vi "Begin.vi"(8 "error in":errorcluster) -> (0 "error out":errorcluster)   [LabVIEW 2018]
doc: "Called before other user functions, this VI is expected to open initial I/O refnums, load in file data, and do all program initialization. Notice that the <B>error out</B> terminal is simply used for data flow. Wiring it to other structures or subVIs ensures that this VI runs first."
uses:
  <vilib>/Rock Robotics/WPI/DriverStation/WPI_DriverStationRobotMode2.ctl
  <vilib>/Rock Robotics/WPI/Joystick/WPI_JoystickDeviceEnum.ctl
  <vilib>/Rock Robotics/SystemInterfaces/DIO/FPGA_DIORelayChannel.ctl
  <vilib>/Rock Robotics/WPI/Relay/WPI_RelayDirection.ctl
  <vilib>/Rock Robotics/SystemInterfaces/AI/FPGA_AIChannel.ctl
  <vilib>/Rock Robotics/SystemInterfaces/DIO/FPGA_DIOChannel.ctl
  GP_states.ctl
  Robot Global Data.vi
  <vilib>/Rock Robotics/Network Tables/NT Write String Array.vi
  <vilib>/Rock Robotics/WPI/RobotDrive/WPI_RobotDriveOpen4MotorWithExistingMotors.vi
  drivers/ADIS16470 IMU/ADIS16470_IMU.lvlib
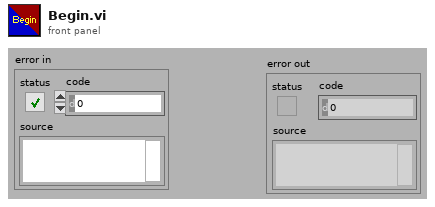
[diagram p1: front panel]
types:
  T1 = typedef "GP_states.ctl" = enum16{"Home", "AutoHome", "Hatch", "Ground"}
  T2 = enum16{"FollowerType_PercentOutput", "FollowerType_AuxOutput1"}
  T3 = typedef "FPGA_DIORelayChannel.ctl" = enum8{"Relay 0", "Relay 1", "Relay 2", "Relay 3", "Invalid"}
  T4 = typedef "WPI_RelayDirection.ctl" = enum16{"Both directions", "Forward only", "Reverse only"}
  T5 = typedef "FPGA_DIOChannel.ctl" = enum8{"DIO 0", "DIO 1", "DIO 2", "DIO 3", "DIO 4", "DIO 5", "DIO 6", "DIO 7", "DIO 8", "DIO 9", "DIO MXP 0", "DIO MXP 1", "DIO MXP 2", "DIO MXP 3", "DIO MXP 4", "DIO MXP 5", "DIO MXP 6", "DIO MXP 7", "DIO MXP 8", "DIO MXP 9", "DIO MXP 10", "DIO MXP 11", "DIO MXP 12", "DIO MXP 13", "DIO MXP 14", "DIO MXP 15", "SPI Port CS1", "SPI Port CS2", "SPI Port CS3", "SPI Port MISO", "SPI Port MOSI", "Invalid"}
  T6 = typedef "FPGA_AIChannel.ctl" = enum8{"AI 0", "AI 1", "AI 2", "AI 3", "AI MXP 0", "AI MXP 1", "AI MXP 2", "AI MXP 3", "Invalid"}
  T7 = typedef "WPI_JoystickDeviceEnum.ctl" = enum16{"USB 0", "USB 1", "USB 2", "USB 3", "USB 4", "USB 5"}
  T8 = typedef "WPI_DriverStationRobotMode2.ctl" = enum16{"Autonomous Disabled", "Autonomous Enabled", "Teleop Disabled", "Teleop Enabled", "Disconnected", "Finish", "Test Disabled", "Test Enabled", "Emergency Stopped"}
  T9 = typedef "WPI_MotorControlDeviceRef.ctl" = cluster{"DeviceStatus":errorcluster, "Type":T10, "PWM":cluster{"PWM Channel":T11, "DeadBand":T12}, "CAN":cluster{"Device Number":u8, "SetOutput VI Ref":variant, "GetOutput VI Ref":variant, "Enable VI Ref":variant, "Disable VI Ref":variant, "Data":variant}, "Invert":bool, "DIO PWM":cluster{"PWM \"Enable\" Channel":T11, "DIOChannel":T5, "PWM Rate":dbl}}
  T10 = typedef "WPI_MotorControlType.ctl" = enum16{"PWM", "CAN", "DIO PWM"}
  T11 = typedef "FPGA_DIOPWMChannel.ctl" = enum8{"PWM 0", "PWM 1", "PWM 2", "PWM 3", "PWM 4", "PWM 5", "PWM 6", "PWM 7", "PWM 8", "PWM 9", "PWM MXP 0", "PWM MXP 1", "PWM MXP 2", "PWM MXP 3", "PWM MXP 4", "PWM MXP 5", "PWM MXP 6", "PWM MXP 7", "PWM MXP 8", "PWM MXP 9", "Invalid"}
  T12 = typedef "WPI_PWMDeadband.ctl" = cluster{"Name":string, "maxPositivePwm":i32, "minPositivePwm":i32, "centerPwm":i32, "maxNegativePwm":i32, "minNegativePwm":i32, "angularRange":u16}
  T13 = typedef "WPI_JoystickDevRef.ctl" = cluster{"Device":T7}
  T14 = typedef "ADIS16470_IMU.lvlib/ADI_IMU_ADIS16470_IMUDevRef.ctl" = cluster{"DevStatus":errorcluster, "Handle":i32, "SPI Bus":T15, "Device Found":bool, "Device Ready":bool, "Serial":u16, "Bytes Per Sample":u16, "Calibrate On Open?":bool}
  T15 = typedef "spi_bus.ctl" = enum16{"SPI On-Board, CS0", "SPI On-Board, CS1", "SPI On-Board, CS2", "SPI On-Board, CS3", "SPI MXP", "Invalid"}
  T16 = typedef "WPI_RobotDriveDevRef.ctl" = cluster{"DevStatus":errorcluster, "Motors[]":T9[], "Square Inputs":bool, "Max Output":dbl}
  T17 = typedef "WPI_RelayDevRef.ctl" = cluster{"DevStatus":errorcluster, "Relay Channel":T3, "Relay Direction":T4}
  T18 = typedef "WPI_PotentiometerDevRef.ctl" = cluster{"DevStatus":errorcluster, "Analog Channel":T6, "Invert Output":bool}
  T19 = typedef "WPI_DigitalInputDevRef.ctl" = cluster{"DevStatus":errorcluster, "DIO Channel":T5}
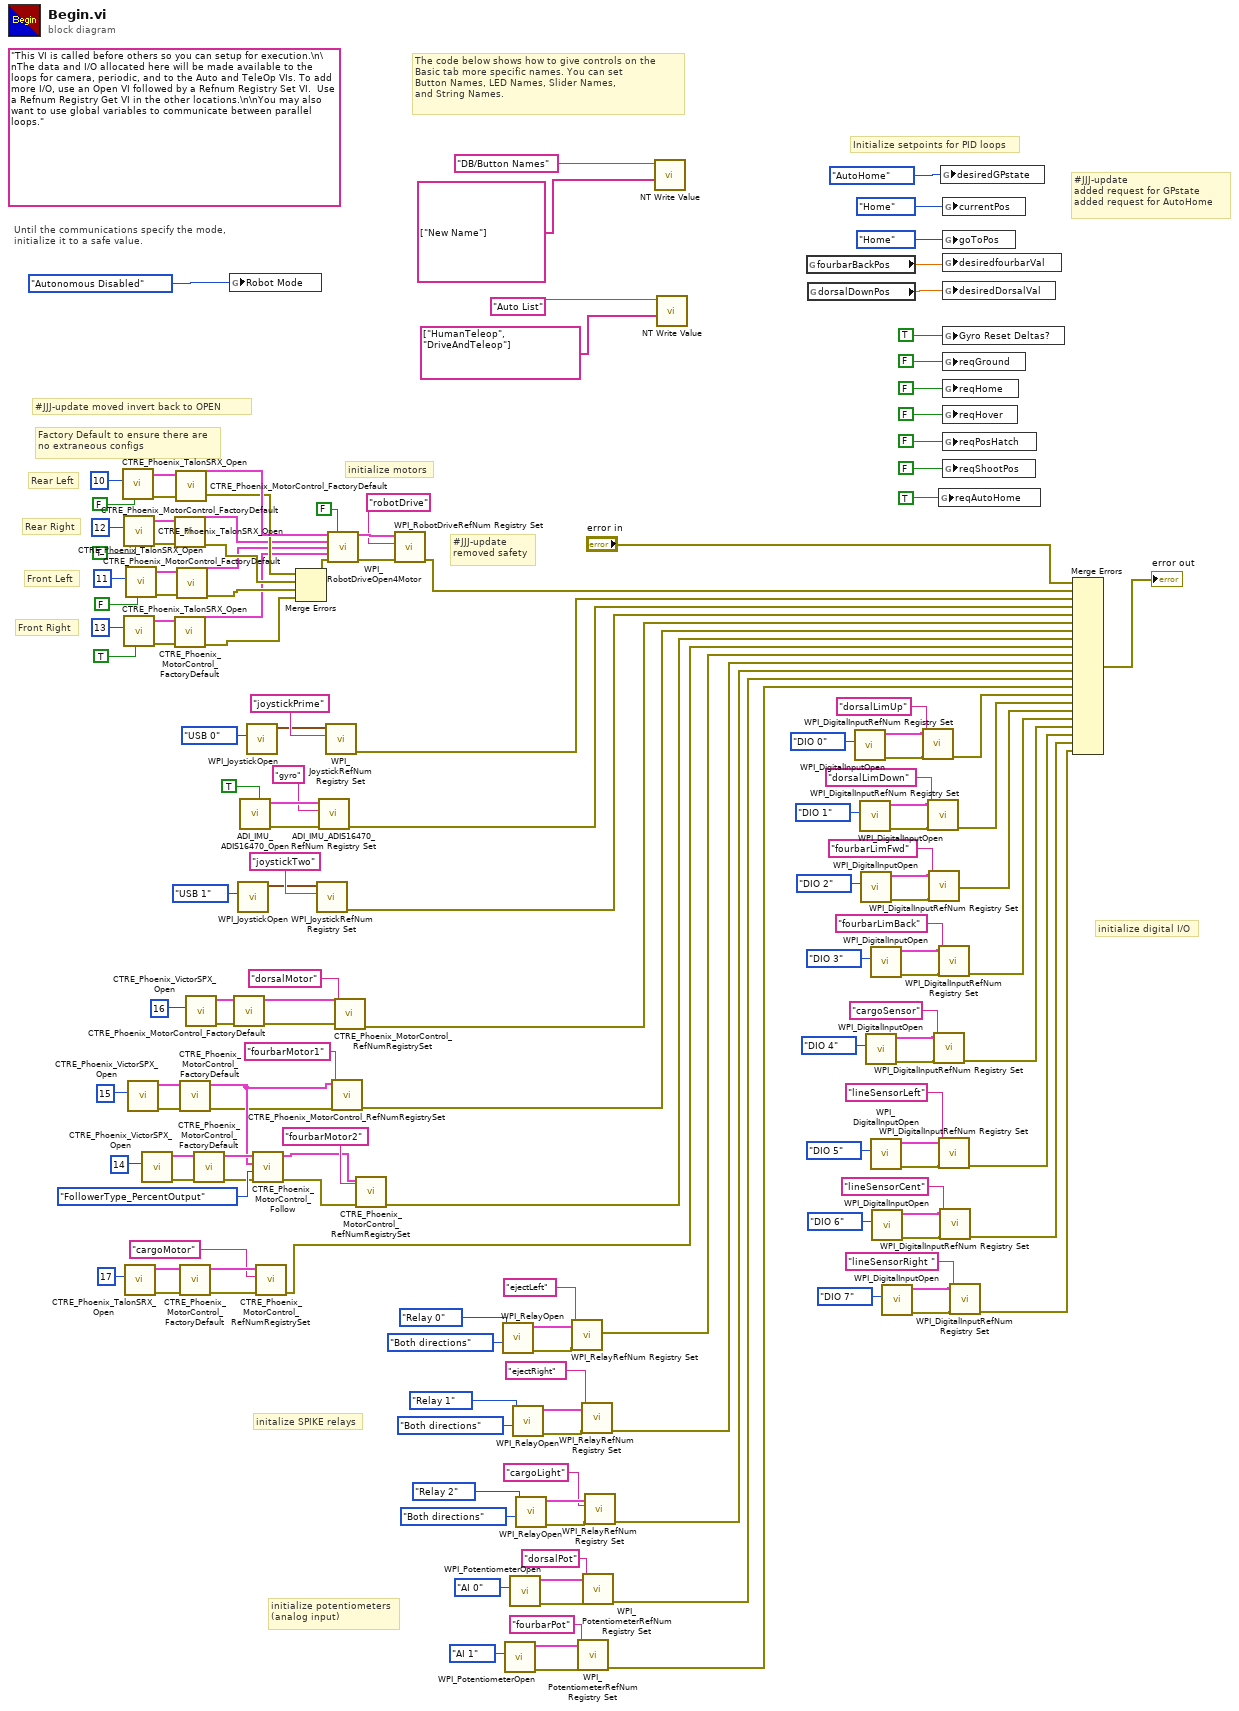
[diagram p0: block diagram]
diagram:
  (unwired) "This VI is called before others so you can setup for execution.\n\nThe data and I/O allocated here will be made available to the loops for camera, periodic, and to the Auto and TeleOp VIs. To add more I/O, use an Open VI followed by a Refnum Registry Set VI.  Use a Refnum Registry Get VI in the other locations.\n\nYou may also want to use global variables to communicate between parallel loops."
  # "#JJJ-update\nadded request for GPstate\nadded request for AutoHome"
  # "#JJJ-update\nremoved safety"
  # "#JJJ-update moved invert back to OPEN"
  # "Initialize setpoints for PID loops"
  # "initialize digital I/O"
  # "initialize potentiometers\n(analog input)"
  # "initalize SPIKE relays"
  # "Factory Default to ensure there are\nno extraneous configs"
  # "Front Right"
  # "Front Left"
  # "Rear Right"
  # "Rear Left"
  # "The code below shows how to give controls on the\nBasic tab more specific names. You can set\nButton Names, LED Names, Slider Names,\nand String Names."
  # "Until the communications specify the mode,\ninitialize it to a safe value."
  # "initialize motors"
  n1 = call <vilib>:"CTRE_Phoenix_TalonSRX_Open.vi"("Invert"=FALSE ("Invert?"), "Device Number"=u8 10) -> ("error out"=w144:errorcluster, "CAN Talon SRX Ref"=w145:T9)  [unwired: 8 in]
  n2 = call <vilib>:"CTRE_Phoenix_TalonSRX_Open.vi"("Invert"=TRUE ("Invert?"), "Device Number"=u8 12) -> ("error out"=w141:errorcluster, "CAN Talon SRX Ref"=w140:T9)  [unwired: 8 in]
  n3 = call <vilib>:"CTRE_Phoenix_TalonSRX_Open.vi"("Invert"=TRUE ("Invert?"), "Device Number"=u8 13) -> ("error out"=w135:errorcluster, "CAN Talon SRX Ref"=w134:T9)  [unwired: 8 in]
  n4 = call <vilib>:"CTRE_Phoenix_TalonSRX_Open.vi"("Device Number"=u8 17) -> ("error out"=w42:errorcluster, "CAN Talon SRX Ref"=w41:T9)  [unwired: 9 in]
  n5 = call <vilib>:"CTRE_Phoenix_TalonSRX_Open.vi"("Invert"=FALSE ("Invert?"), "Device Number"=u8 11) -> ("error out"=w136:errorcluster, "CAN Talon SRX Ref"=w137:T9)  [unwired: 8 in]
  n6 = call <vilib>:"CTRE_Phoenix_VictorSPX_Open.vi"("Device Number"=u8 15) -> ("error out"=w39:errorcluster, "CAN Talon SRX Ref"=w117:T9)  [unwired: 9 in]
  n7 = call <vilib>:"CTRE_Phoenix_VictorSPX_Open.vi"("Device Number"=u8 14) -> ("error out"=w40:errorcluster, "CAN Talon SRX Ref"=w114:T9)  [unwired: 9 in]
  n8 = call <vilib>:"CTRE_Phoenix_MotorControl_FactoryDefault.vi"("error in"=w141, "PhoenixMotorControlDevRef"=w140) -> ("error out"=w7:errorcluster, "PhoenixMotorControlDevRef"=w8:T9)  [unwired: 8 in]
  n9 = call <vilib>:"CTRE_Phoenix_MotorControl_FactoryDefault.vi"("error in"=w135, "PhoenixMotorControlDevRef"=w134) -> ("error out"=w3:errorcluster, "PhoenixMotorControlDevRef"=w4:T9)  [unwired: 8 in]
  n10 = call <vilib>:"CTRE_Phoenix_MotorControl_FactoryDefault.vi"("error in"=w144, "PhoenixMotorControlDevRef"=w145) -> ("error out"=w9:errorcluster, "PhoenixMotorControlDevRef"=w10:T9)  [unwired: 8 in]
  n11 = call <vilib>:"CTRE_Phoenix_MotorControl_FactoryDefault.vi"("error in"=w136, "PhoenixMotorControlDevRef"=w137) -> ("error out"=w5:errorcluster, "PhoenixMotorControlDevRef"=w6:T9)  [unwired: 8 in]
  n12 = call <vilib>:"CTRE_Phoenix_MotorControl_FactoryDefault.vi"("error in"=w39, "PhoenixMotorControlDevRef"=w117) -> ("error out"=w26:errorcluster, "PhoenixMotorControlDevRef"=w27:T9)  [unwired: 8 in]
  n13 = call <vilib>:"CTRE_Phoenix_MotorControl_FactoryDefault.vi"("error in"=w42, "PhoenixMotorControlDevRef"=w41) -> ("error out"=w36:errorcluster, "PhoenixMotorControlDevRef"=w37:T9)  [unwired: 8 in]
  n14 = call <vilib>:"CTRE_Phoenix_VictorSPX_Open.vi"("Device Number"=u8 16) -> ("error out"=w38:errorcluster, "CAN Talon SRX Ref"=w120:T9)  [unwired: 9 in]
  n15 = call <vilib>:"CTRE_Phoenix_MotorControl_FactoryDefault.vi"("error in"=w40, "PhoenixMotorControlDevRef"=w114) -> ("error out"=w31:errorcluster, "PhoenixMotorControlDevRef"=w33:T9)  [unwired: 8 in]
  n16 = global write "Robot Global Data.vi" "Robot Mode"(WPI_DriverStationRobotMode2."Autonomous Disabled" ("Robot Mode")) -> ()
  n17 = call <vilib>:"CTRE_Phoenix_MotorControl_FactoryDefault.vi"("error in"=w38, "PhoenixMotorControlDevRef"=w120) -> ("error out"=w28:errorcluster, "PhoenixMotorControlDevRef"=w29:T9)  [unwired: 8 in]
  n18 = call <vilib>:"WPI_JoystickOpen.vi"("JoystickDevice"=WPI_JoystickDeviceEnum."USB 1") -> ("JoystickDevRef"=w125:T13)  [unwired: 10 in]
  n19 = call "ADI_IMU_ADIS16470_Open.vi"("Calibrate On Open"=TRUE) -> ("error out"=w131:errorcluster, "ADI IMU DevRef Out"=w130:T14)  [unwired: 9 in]
  n20 = call <vilib>:"WPI_JoystickOpen.vi"("JoystickDevice"=WPI_JoystickDeviceEnum."USB 0") -> ("JoystickDevRef"=w156:T13)  [unwired: 10 in]
  n21 = call <vilib>:"CTRE_Phoenix_MotorControl_Follow.vi"("error in (no error)"=w31, "FollowerType"=T2."FollowerType_PercentOutput", "Master Controller to Follow"=w27, "PhoenixMotorControlDevRef"=w33) -> ("error out"=w24:errorcluster, "PhoenixMotorControlDevRef"=w25:T9)  [unwired: 6 in]
  n22 = call <vilib>:"CTRE_Phoenix_MotorControl_RefNumRegistrySet.vi"("error in (no error)"=w36, "refnum name"="cargoMotor", "PhoenixMotorControlDevRef"=w37) -> ("error out"=w30:errorcluster)  [unwired: 7 in, 1 out]
  n23 = Merge Errors(w9, w7, w5, w3) -> (w143:errorcluster)
  n24 = call <vilib>:"WPI_JoystickRefNum Registry Set.vi"("refnum name"="joystickTwo", "JoystickDevRef"=w125) -> ("error out"=w123:errorcluster)  [unwired: 8 in, 1 out]
  n25 = call "ADI_IMU_ADIS16470_RefNum Registry Set.vi"("error in (no error)"=w131, "refnum name"="gyro", "ADI IMU DevRef"=w130) -> ("error out"=w128:errorcluster)  [unwired: 7 in, 1 out]
  n26 = call <vilib>:"WPI_JoystickRefNum Registry Set.vi"("refnum name"="joystickPrime", "JoystickDevRef"=w156) -> ("error out"=w149:errorcluster)  [unwired: 8 in, 1 out]
  n27 = call-poly <vilib>:"WPI_RobotDriveOpen4Motor.vi"("Rear Left Motor Dev Ref"=w10, "Square Inputs"=FALSE, "Rear Right Motor Dev Ref"=w8, "Front Left Motor Dev Ref"=w6, "Front Right Motor Dev Ref"=w4, "error in (no error)"=w143) -> ("RobotDriveDevRef"=w161:T16, "error out"=w159:errorcluster)  [unwired: 8 in]
  n28 = call <vilib>:"CTRE_Phoenix_MotorControl_RefNumRegistrySet.vi"("error in (no error)"=w26, "refnum name"="fourbarMotor1", "PhoenixMotorControlDevRef"=w27) -> ("error out"=w112:errorcluster)  [unwired: 7 in, 1 out]
  n29 = call <vilib>:"CTRE_Phoenix_MotorControl_RefNumRegistrySet.vi"("error in (no error)"=w28, "refnum name"="dorsalMotor", "PhoenixMotorControlDevRef"=w29) -> ("error out"=w121:errorcluster)  [unwired: 7 in, 1 out]
  n30 = call <vilib>:"CTRE_Phoenix_MotorControl_RefNumRegistrySet.vi"("error in (no error)"=w24, "refnum name"="fourbarMotor2", "PhoenixMotorControlDevRef"=w25) -> ("error out"=w111:errorcluster)  [unwired: 7 in, 1 out]
  n31 = call <vilib>:"WPI_RobotDriveRefNum Registry Set.vi"("error in (no error)"=w159, "refnum name"="robotDrive", "RobotDriveDevRef"=w161) -> ("error out"=w146:errorcluster)  [unwired: 1 in, 7 out]
  n32 = call <vilib>:"WPI_RelayOpen.vi"("Relay Direction"=WPI_RelayDirection."Both directions", "Relay Channel"=FPGA_DIORelayChannel."Relay 0") -> ("error out"=w109:errorcluster, "RelayDevRef"=w110:T17)  [unwired: 8 in]
  n33 = call <vilib>:"WPI_PotentiometerOpen.vi"("Analog Channel"=FPGA_AIChannel."AI 1") -> ("error out"=w91:errorcluster, "PotDevRef"=w94:T18)  [unwired: 9 in]
  n34 = call <vilib>:"WPI_PotentiometerOpen.vi"("Analog Channel"=FPGA_AIChannel."AI 0") -> ("error out"=w95:errorcluster, "PotDevRef"=w98:T18)  [unwired: 9 in]
  n35 = call <vilib>:"WPI_RelayOpen.vi"("Relay Direction"=WPI_RelayDirection."Both directions", "Relay Channel"=FPGA_DIORelayChannel."Relay 1") -> ("error out"=w104:errorcluster, "RelayDevRef"=w105:T17)  [unwired: 8 in]
  n36 = call <vilib>:"WPI_RelayOpen.vi"("Relay Direction"=WPI_RelayDirection."Both directions", "Relay Channel"=FPGA_DIORelayChannel."Relay 2") -> ("error out"=w46:errorcluster, "RelayDevRef"=w45:T17)  [unwired: 8 in]
  n37 = call <vilib>:"WPI_RelayRefNum Registry Set.vi"("error in (no error)"=w109, "refnum name"="ejectLeft", "RelayDevRef"=w110) -> ("error out"=w100:errorcluster)  [unwired: 7 in, 1 out]
  n38 = call <vilib>:"WPI_PotentiometerRefNum Registry Set.vi"("error in (no error)"=w91, "refnum name"="fourbarPot", "PotDevRef"=w94) -> ("error out"=w89:errorcluster)  [unwired: 7 in, 1 out]
  n39 = call <vilib>:"WPI_RelayRefNum Registry Set.vi"("error in (no error)"=w104, "refnum name"="ejectRight", "RelayDevRef"=w105) -> ("error out"=w99:errorcluster)  [unwired: 7 in, 1 out]
  n40 = call <vilib>:"WPI_PotentiometerRefNum Registry Set.vi"("error in (no error)"=w95, "refnum name"="dorsalPot", "PotDevRef"=w98) -> ("error out"=w90:errorcluster)  [unwired: 7 in, 1 out]
  n41 = call <vilib>:"WPI_RelayRefNum Registry Set.vi"("error in (no error)"=w46, "refnum name"="cargoLight", "RelayDevRef"=w45) -> ("error out"=w43:errorcluster)  [unwired: 7 in, 1 out]
  n42 = call-poly <vilib>:"NT Write Value.vi"("String Array"=string[] ["New Name"], "Name"="DB/Button Names") -> ()  [unwired: 9 in, 1 out]
  n43 = call-poly <vilib>:"NT Write Value.vi"("String Array"=string[] ["HumanTeleop", "DriveAndTeleop"], "Name"="Auto List") -> ()  [unwired: 9 in, 1 out]
  n44 = global read "Robot Global Data.vi" "fourbarBackPos"() -> (w15:dbl)
  n45 = global read "Robot Global Data.vi" "dorsalDownPos"() -> (w16:dbl)
  n46 = call <vilib>:"WPI_DigitalInputOpen.vi"("DIO Channel"=FPGA_DIOChannel."DIO 0") -> ("error out"=w86:errorcluster, "DigitalInputDevRef"=w88:T19)  [unwired: 9 in]
  n47 = call <vilib>:"WPI_DigitalInputOpen.vi"("DIO Channel"=FPGA_DIOChannel."DIO 1") -> ("error out"=w83:errorcluster, "DigitalInputDevRef"=w85:T19)  [unwired: 9 in]
  n48 = call <vilib>:"WPI_DigitalInputOpen.vi"("DIO Channel"=FPGA_DIOChannel."DIO 2") -> ("error out"=w80:errorcluster, "DigitalInputDevRef"=w82:T19)  [unwired: 9 in]
  n49 = call <vilib>:"WPI_DigitalInputOpen.vi"("DIO Channel"=FPGA_DIOChannel."DIO 4") -> ("error out"=w70:errorcluster, "DigitalInputDevRef"=w72:T19)  [unwired: 9 in]
  n50 = call <vilib>:"WPI_DigitalInputOpen.vi"("DIO Channel"=FPGA_DIOChannel."DIO 3") -> ("error out"=w77:errorcluster, "DigitalInputDevRef"=w79:T19)  [unwired: 9 in]
  n51 = call <vilib>:"WPI_DigitalInputOpen.vi"("DIO Channel"=FPGA_DIOChannel."DIO 5") -> ("error out"=w67:errorcluster, "DigitalInputDevRef"=w69:T19)  [unwired: 9 in]
  n52 = call <vilib>:"WPI_DigitalInputOpen.vi"("DIO Channel"=FPGA_DIOChannel."DIO 6") -> ("error out"=w64:errorcluster, "DigitalInputDevRef"=w66:T19)  [unwired: 9 in]
  n53 = call <vilib>:"WPI_DigitalInputOpen.vi"("DIO Channel"=FPGA_DIOChannel."DIO 7") -> ("error out"=w61:errorcluster, "DigitalInputDevRef"=w63:T19)  [unwired: 9 in]
  n54 = call <vilib>:"WPI_DigitalInputRefNum Registry Set.vi"("error in (no error)"=w86, "refnum name"="dorsalLimUp", "DigitalInputDevRef"=w88) -> ("error out"=w56:errorcluster)  [unwired: 7 in, 1 out]
  n55 = call <vilib>:"WPI_DigitalInputRefNum Registry Set.vi"("error in (no error)"=w83, "refnum name"="dorsalLimDown", "DigitalInputDevRef"=w85) -> ("error out"=w55:errorcluster)  [unwired: 7 in, 1 out]
  n56 = call <vilib>:"WPI_DigitalInputRefNum Registry Set.vi"("error in (no error)"=w80, "refnum name"="fourbarLimFwd", "DigitalInputDevRef"=w82) -> ("error out"=w54:errorcluster)  [unwired: 7 in, 1 out]
  n57 = call <vilib>:"WPI_DigitalInputRefNum Registry Set.vi"("error in (no error)"=w70, "refnum name"="cargoSensor", "DigitalInputDevRef"=w72) -> ("error out"=w52:errorcluster)  [unwired: 7 in, 1 out]
  n58 = global write "Robot Global Data.vi" "reqAutoHome"(TRUE ("reqGround")) -> ()
  n59 = call <vilib>:"WPI_DigitalInputRefNum Registry Set.vi"("error in (no error)"=w77, "refnum name"="fourbarLimBack", "DigitalInputDevRef"=w79) -> ("error out"=w53:errorcluster)  [unwired: 7 in, 1 out]
  n60 = call <vilib>:"WPI_DigitalInputRefNum Registry Set.vi"("error in (no error)"=w67, "refnum name"="lineSensorLeft", "DigitalInputDevRef"=w69) -> ("error out"=w51:errorcluster)  [unwired: 7 in, 1 out]
  n61 = call <vilib>:"WPI_DigitalInputRefNum Registry Set.vi"("error in (no error)"=w64, "refnum name"="lineSensorCent", "DigitalInputDevRef"=w66) -> ("error out"=w50:errorcluster)  [unwired: 7 in, 1 out]
  n62 = global write "Robot Global Data.vi" "desiredGPstate"(GP_states."AutoHome" ("currentPos")) -> ()
  n63 = global write "Robot Global Data.vi" "currentPos"(GP_states."Home" ("currentPos")) -> ()
  n64 = global write "Robot Global Data.vi" "goToPos"(GP_states."Home" ("currentPos")) -> ()
  n65 = global write "Robot Global Data.vi" "desiredfourbarVal"(w15) -> ()
  n66 = global write "Robot Global Data.vi" "desiredDorsalVal"(w16) -> ()
  n67 = global write "Robot Global Data.vi" "Gyro Reset Deltas?"(TRUE) -> ()
  n68 = global write "Robot Global Data.vi" "reqGround"(FALSE ("reqGround")) -> ()
  n69 = global write "Robot Global Data.vi" "reqHome"(FALSE ("reqGround")) -> ()
  n70 = global write "Robot Global Data.vi" "reqHover"(FALSE ("reqGround")) -> ()
  n71 = global write "Robot Global Data.vi" "reqPosHatch"(FALSE ("reqGround")) -> ()
  n72 = global write "Robot Global Data.vi" "reqShootPos"(FALSE ("reqGround")) -> ()
  n73 = call <vilib>:"WPI_DigitalInputRefNum Registry Set.vi"("error in (no error)"=w61, "refnum name"="lineSensorRight ", "DigitalInputDevRef"=w63) -> ("error out"=w49:errorcluster)  [unwired: 7 in, 1 out]
  n74 = Merge Errors("error in", w146, w149, w128, w123, w121, w112, w111, w30, w100, w99, w43, w90, w89, w56, w55, w54, w53, w52, w51, w50, w49) -> (→"error out":errorcluster)
